vi "BusRatio.vi"() -> ()   [LabVIEW 2017]
uses:
  globe.vi
panel:
  out "总线利用率(%)":dbl
  in  "采样周期（ms）":u32(slide)=200 min=200 max=2000 step=100 scale=200.0..2000.0
  out "总线利用率波形图表":dbl(graph)
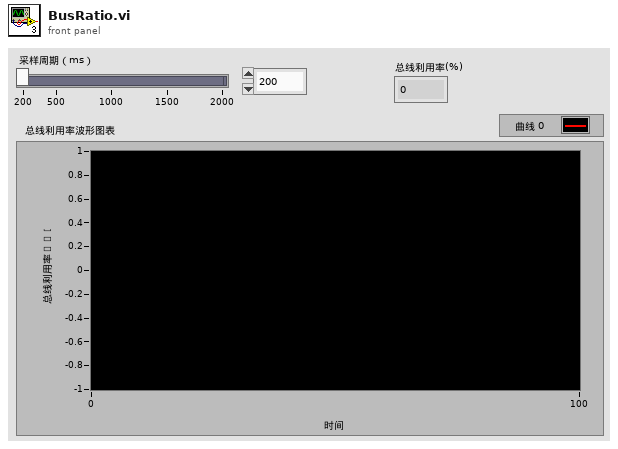
[diagram p1: front panel]
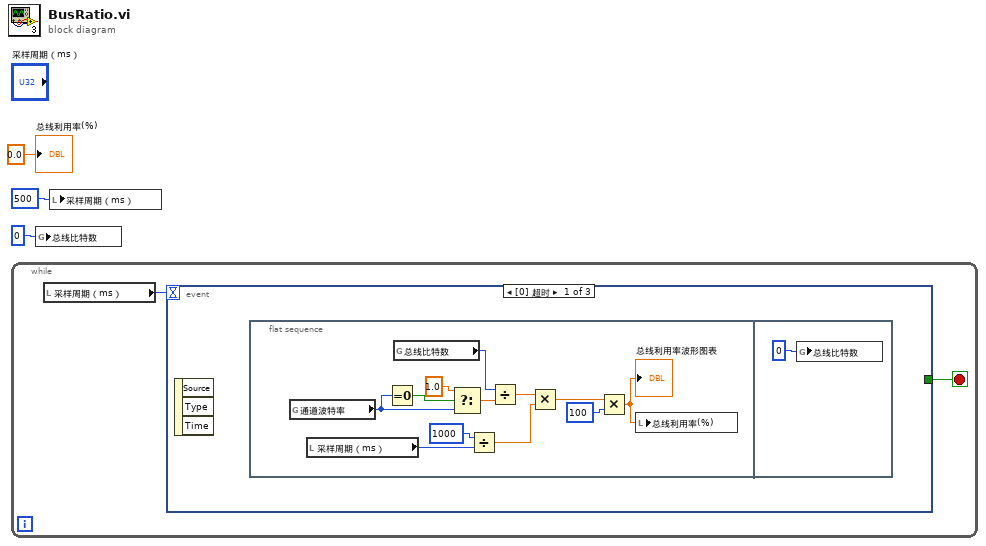
[diagram p0: block diagram]
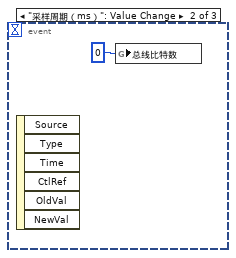
[diagram p2: hidden frame]
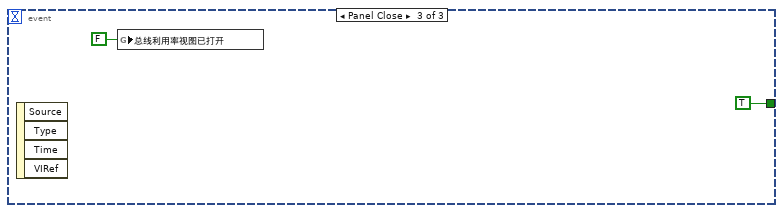
[diagram p3: hidden frame]
diagram:
  n1 = while {
    stop <- w5 stop-if-true
    n2 = local read "采样周期（ms）"() -> (w4:u32)
    n3 = event shown="[0] 超时" {
      selector: _ -> [_ _ _]
      dyn-events: _ -> [_ _ _]
      timeout: w4 -> [_ _ _]
      tunnel: [_ _ TRUE] -> w5
      event Timeout {
        n4 = event-data() -> ()  [unwired: 1 in, 3 out]
        n5 = flat-sequence {
          frame #0 {
            n6 = global read "globe.vi" "通道波特率"() -> (w8:u32)
            n7 = local read "采样周期（ms）"() -> (w15:u32)
            n8 = Equal To 0?(x=w8) -> (x = 0?=w10:bool)
            n9 = global read "globe.vi" "总线比特数"() -> (w17:u64)
            n10 = Select(t=1.0, s=w10, f=w8) -> (s? t:f=w7:dbl)
            n11 = Divide(x=1000, y=w15) -> (x/y=w13:dbl)
            n12 = Divide(x=w17, y=w7) -> (x/y=w14:dbl)
            n13 = Multiply(x=w14, y=w13) -> (x*y=w12:dbl)
            n14 = Multiply(x=w12, y=100) -> (x*y=w6:dbl)
            "总线利用率波形图表" <- w6
            n15 = local write "总线利用率(%)"(w6) -> ()
          }
          frame #1 {
            n16 = global write "globe.vi" "总线比特数"(u64 0 ("总线比特数")) -> ()
          }
        }
      }
      event "采样周期（ms）": Value Change {
        n17 = event-data() -> ()  [unwired: 1 in, 6 out]
        n18 = global write "globe.vi" "总线比特数"(u64 0 ("总线比特数")) -> ()
      }
      event Panel Close {
        n19 = event-data() -> ()  [unwired: 1 in, 4 out]
        n20 = global write "globe.vi" "总线利用率视图已打开"(FALSE) -> ()
      }
    }
  }
  n21 = global write "globe.vi" "总线比特数"(u64 0 ("总线比特数")) -> ()
  n22 = local write "采样周期（ms）"(u32 500 ("采样周期（ms）")) -> ()
  "总线利用率(%)" <- 0.0 ("总线利用率(%)")
